vi "Create Library Folder.vi"(11 "Script Strategy in":refnum<class "Script Strategy.lvclass">) -> (2 "Library Folder Already Exists?":bool, 3 "Script Strategy out":refnum<class "Script Strategy.lvclass">)   [LabVIEW 2021, in "_Create From Template.lvlib" / "Script Strategy.lvlib" / "Script Strategy.lvclass"]
uses:
  Script Strategy.lvclass
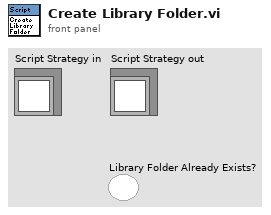
[diagram p1: front panel]
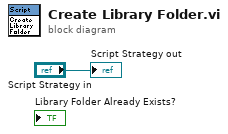
[diagram p0: block diagram]
diagram:
  "Script Strategy out" <- "Script Strategy in"
